vi "Read Maximum.vi"(8 "error in (no error)":errorcluster, 11 "VISA resource name":refnum<visa-resource-name>) -> (0 "error out":errorcluster, 1 "MAX Current":dbl, 2 "MAX Voltage":dbl, 3 "VISA resource name out":refnum<visa-resource-name>)   [LabVIEW 2021, in "BK Precision 169XB.lvlib"]
doc: "Returns the actual voltage level and actual current level for a desired channel."
uses:
  BK Precision 169XB.lvlib
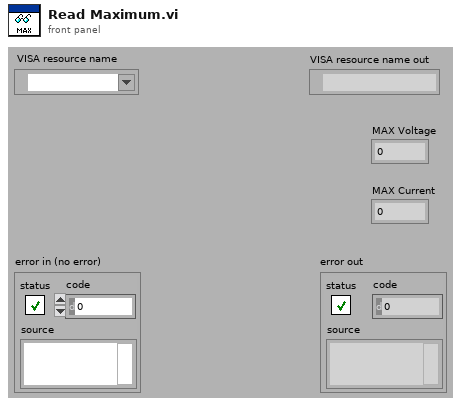
[diagram p1: front panel]
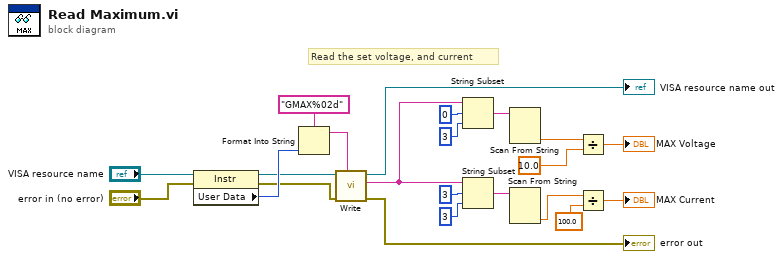
[diagram p0: block diagram]
diagram:
  # "Read the set voltage, and current"
  n1 = property class="Instr"(reference="VISA resource name", error in="error in (no error)") -> (reference out=w5:refnum<visa-resource-name>, error out=w4:errorcluster, "User Data"=w7:u32)
  n2 = Format Into String(format string="GMAX%02d", w7) -> (resulting string=w2:string)  [unwired: 2 in, 1 out]
  n3 = call "Write.vi"("Input String"=w2, "error in (no error)"=w4, "VISA resource name"=w5) -> ("error out"=→"error out":errorcluster, "String"=w15:string, "VISA resource name out"=→"VISA resource name out":refnum<visa-resource-name>)  [unwired: 6 in]
  n4 = String Subset(string=w15, offset (0)=0, length (rest)=3 ("length (rest)")) -> (substring=w21:string)
  n5 = String Subset(string=w15, offset (0)=3, length (rest)=3 ("length (rest)")) -> (substring=w20:string)
  n6 = Scan From String(input string=w21) -> (output 1=w17:dbl)  [unwired: 4 in, 3 out]
  n7 = Scan From String(input string=w20) -> (output 1=w14:dbl)  [unwired: 4 in, 3 out]
  n8 = Divide(x=w17, y=10.0) -> (x/y=→"MAX Voltage":dbl)
  n9 = Divide(x=w14, y=100.0) -> (x/y=→"MAX Current":dbl)
